vi "Get Parent.vi"(8 "error in (no error)":errorcluster, 11 "NodeRef In":refnum<data-value>) -> (0 "error out":errorcluster, 2 "Parent":refnum<data-value>, 3 "NodeRef":refnum<data-value>)   [LabVIEW 2020, in "PicoG-ParserLexer.lvlib" / "Node.lvclass"]
doc: "Gets the parent of this node. Will return NotARef if there is no parent which can mean this node is the root or not currently in the tree.\n\n<b>Error Codes:</b>\n<b>1556</b>: Node not instantiated. Nodes must be initialized with Ctor first."
uses:
  Node.lvclass
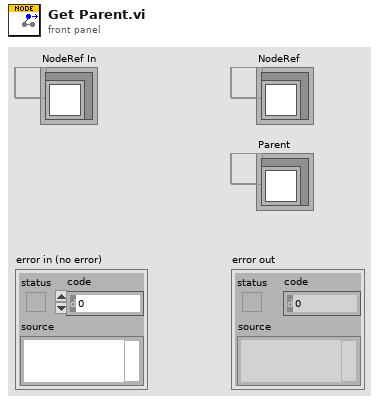
[diagram p1: front panel]
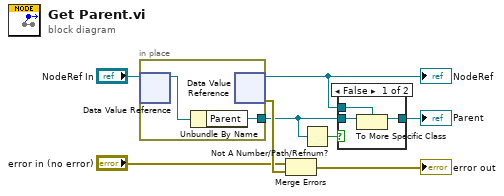
[diagram p0: block diagram]
diagram:
  n1 = in-place {
    in-place-border: [w9] -> w4
    n2 = in-place-dvr #1("NodeRef In") -> (w10:refnum<class "Node.lvclass">)  [unwired: 1 out]
    n3 = Unbundle By Name(w10) -> ("Parent"=w9:refnum<data-value>)
    n4 = in-place-dvr #1() -> (w3:refnum<data-value>, w8:errorcluster)  [unwired: 1 in]
  }
  "NodeRef" <- w3
  n5 = Merge Errors("error in (no error)", w8) -> (→"error out":errorcluster)
  n6 = Not A Number/Path/Refnum?(number/path/refnum=w4) -> (NaN/Path/Refnum?=w5:bool)
  n7 = case shown="False" w5 {
    tunnel: w4 -> [w13 _]
    tunnel: w3 -> [w12 _]
    tunnel: [w11 _] -> w2
    frame False {
      n8 = To More Specific Class(target class=w12, reference=w13) -> (specific class reference=w11:refnum<data-value>)  [unwired: 1 in, 1 out]
    }
    frame True {
    }
  }
  "Parent" <- w2
